vi "6_4.vi"   [LabVIEW 2017]
uses:
  <vilib>/Utility/file.llb/Write Delimited Spreadsheet (DBL).vi
  <vilib>/measure/NI_MABase.lvlib
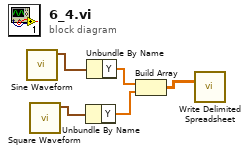
[diagram p0: block diagram]
diagram:
  n1 = call <vilib>:"Sine Waveform.vi"() -> ("signal out"=w2:waveform(dbl))  [unwired: 10 in, 1 out]
  n2 = call <vilib>:"Square Waveform.vi"() -> ("signal out"=w1:waveform(dbl))  [unwired: 10 in, 1 out]
  n3 = Unbundle By Name(w1) -> ("Y"=w3:dbl[])
  n4 = Unbundle By Name(w2) -> ("Y"=w4:dbl[])
  n5 = Build Array(w4, w3) -> (w5:dbl[][])
  n6 = call-poly <vilib>:"Write Delimited Spreadsheet.vi"("2D data"=w5) -> ()  [unwired: 13 in, 2 out]
